vi "SQL_table_users_admin_select_table.vi"() -> (0 "error out":errorcluster, 1 "管理员个数":i32, 3 "管理员信息":string[][](table))   [LabVIEW 2014]
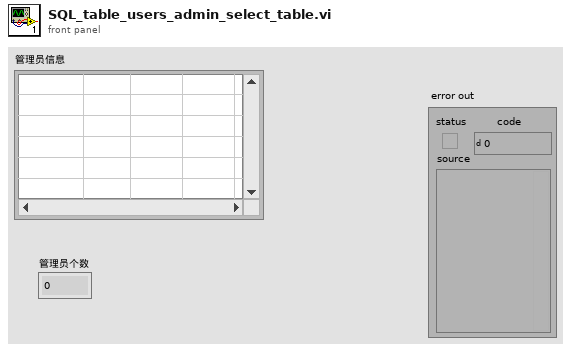
[diagram p1: front panel]
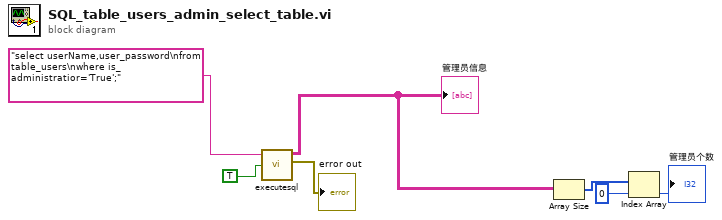
[diagram p0: block diagram]
diagram:
  n1 = call "executesql.vi"("Return Data (T)"=TRUE, "Command Text"="select userName,user_password\nfrom table_users\nwhere is_administratior='True';") -> ("error out"=→"error out":errorcluster, "Data"=w4:string[][])  [unwired: 5 in]
  "管理员信息" <- w4
  n2 = Array Size(array=w4) -> (size(s)=w3:i32[])
  n3 = Index Array(array=w3, index=0) -> (element=→"管理员个数":i32)
